vi "PM5000_VIF_demo_G2.vi"(2 "error in (no error)":errorcluster) -> (0 "error out":errorcluster, 1 "VIF_cluster":T1)   [LabVIEW 2018]
uses:
  Controls/VIF_cluster.ctl
panel:
  in  "Variacion Frecuencia":sgl=0.1
  in  "Variacion Voltaje":sgl=5.0
  in  "Frec_AVG":dbl=60.0
  in  "Frec.":dbl=60.0
  in  "I3":dbl=325.0
  in  "I2":dbl=320.0
  in  "I1":dbl=350.0
  in  "V3_V1":dbl=450.0
  in  "V2_V3":dbl=450.0
  in  "V1_V2":dbl=450.0
  # "VOLTAJES"
  # "CORRIENTE"
  # "FRECUENCIA"
  # "G02"
  # "G02"
  # "G02"
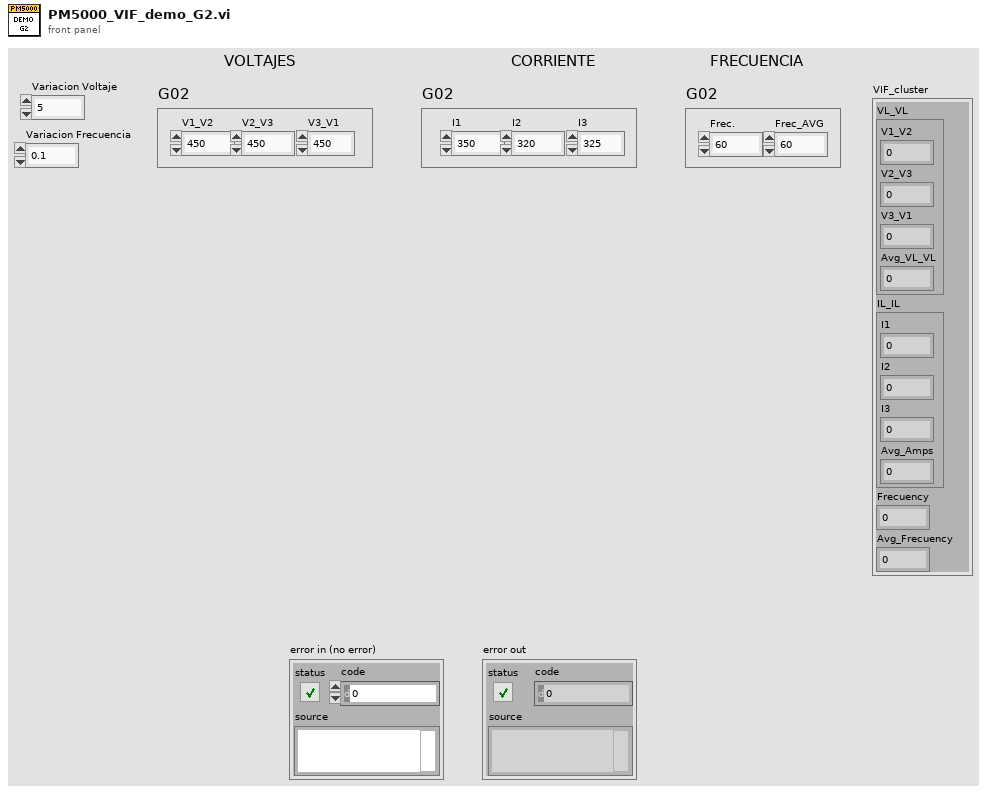
[diagram p1: front panel]
types:
  T1 = typedef "VIF_cluster.ctl" = cluster{"VL_VL":cluster{"V1_V2":sgl, "V2_V3":sgl, "V3_V1":sgl, "Avg_VL_VL":sgl}, "IL_IL":cluster{"I1":sgl, "I2":sgl, "I3":sgl, "Avg_Amps":sgl}, "Frecuency":sgl, "Avg_Frecuency":sgl}
  T2 = cluster{"I1 (A)":sgl, "I2 (A)":sgl, "I3 (A)":sgl, "Avg_Amps":sgl}
  T3 = cluster{"V1_V2 (V)":sgl, "V2_V3 (V)":sgl, "V3_V1 (V)":sgl, "Avg_VL_VL":sgl}
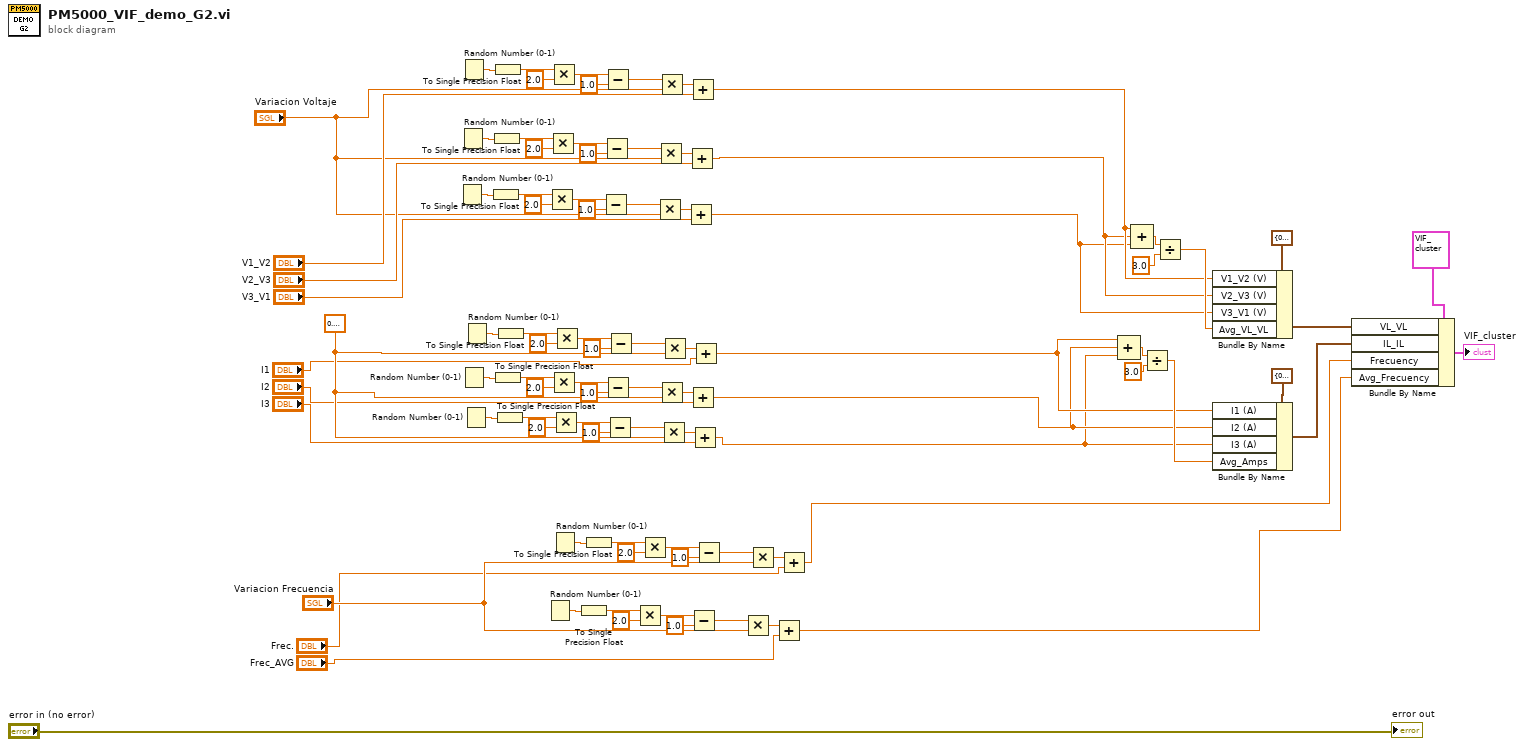
[diagram p0: block diagram]
diagram:
  w26 = sgl 0.1 ("y")
  n1 = Random Number (0-1)() -> (number: 0 to 1=w56:dbl)
  n2 = Random Number (0-1)() -> (number: 0 to 1=w64:dbl)
  n3 = Random Number (0-1)() -> (number: 0 to 1=w72:dbl)
  n4 = Random Number (0-1)() -> (number: 0 to 1=w37:dbl)
  n5 = Random Number (0-1)() -> (number: 0 to 1=w30:dbl)
  n6 = Random Number (0-1)() -> (number: 0 to 1=w44:dbl)
  n7 = To Single Precision Float(number=w56) -> (single precision float=w55:sgl)
  n8 = To Single Precision Float(number=w64) -> (single precision float=w65:sgl)
  n9 = To Single Precision Float(number=w72) -> (single precision float=w71:sgl)
  n10 = To Single Precision Float(number=w37) -> (single precision float=w36:sgl)
  n11 = To Single Precision Float(number=w30) -> (single precision float=w31:sgl)
  n12 = To Single Precision Float(number=w44) -> (single precision float=w45:sgl)
  n13 = Random Number (0-1)() -> (number: 0 to 1=w9:dbl)
  n14 = Multiply(x=w55, y=sgl 2.0) -> (x*y=w58:sgl)
  n15 = Multiply(x=w65, y=sgl 2.0) -> (x*y=w62:sgl)
  n16 = Multiply(x=w71, y=sgl 2.0) -> (x*y=w74:sgl)
  n17 = Multiply(x=w36, y=sgl 2.0) -> (x*y=w39:sgl)
  n18 = Random Number (0-1)() -> (number: 0 to 1=w16:dbl)
  n19 = Multiply(x=w31, y=sgl 2.0) -> (x*y=w28:sgl)
  n20 = Multiply(x=w45, y=sgl 2.0) -> (x*y=w42:sgl)
  n21 = To Single Precision Float(number=w9) -> (single precision float=w10:sgl)
  n22 = To Single Precision Float(number=w16) -> (single precision float=w15:sgl)
  n23 = Subtract(x=w58, y=sgl 1.0) -> (x-y=w54:sgl)
  n24 = Subtract(x=w62, y=sgl 1.0) -> (x-y=w66:sgl)
  n25 = Subtract(x=w74, y=sgl 1.0) -> (x-y=w70:sgl)
  n26 = Subtract(x=w39, y=sgl 1.0) -> (x-y=w35:sgl)
  n27 = Subtract(x=w28, y=sgl 1.0) -> (x-y=w32:sgl)
  n28 = Subtract(x=w42, y=sgl 1.0) -> (x-y=w46:sgl)
  n29 = Multiply(x=w10, y=sgl 2.0) -> (x*y=w7:sgl)
  n30 = Multiply(x=w15, y=sgl 2.0) -> (x*y=w18:sgl)
  n31 = Multiply(x=w54, y="Variacion Voltaje") -> (x*y=w53:sgl)
  n32 = Multiply(x=w66, y="Variacion Voltaje") -> (x*y=w67:sgl)
  n33 = Multiply(x=w70, y="Variacion Voltaje") -> (x*y=w69:sgl)
  n34 = Multiply(x=w35, y=w26) -> (x*y=w34:sgl)
  n35 = Multiply(x=w32, y=w26) -> (x*y=w33:sgl)
  n36 = Multiply(x=w46, y=w26) -> (x*y=w47:sgl)
  n37 = Add(x=w53, y="V3_V1") -> (x+y=w48:dbl)
  n38 = Add(x=w67, y="V2_V3") -> (x+y=w49:dbl)
  n39 = Add(x=w69, y="V1_V2") -> (x+y=w50:dbl)
  n40 = Add(x=w34, y="I2") -> (x+y=w21:dbl)
  n41 = Subtract(x=w7, y=sgl 1.0) -> (x-y=w11:sgl)
  n42 = Add(x=w33, y="I3") -> (x+y=w20:dbl)
  n43 = Add(x=w47, y="I1") -> (x+y=w22:dbl)
  n44 = Subtract(x=w18, y=sgl 1.0) -> (x-y=w14:sgl)
  n45 = Multiply(x=w11, y="Variacion Frecuencia") -> (x*y=w12:sgl)
  n46 = Multiply(x=w14, y="Variacion Frecuencia") -> (x*y=w13:sgl)
  n47 = Add(x=w12, y="Frec_AVG") -> (x+y=w3:dbl)
  n48 = Add(x=w13, y="Frec.") -> (x+y=w4:dbl)
  n49 = Compound Arithmetic op=ADD(w22, w21, w20) -> (w77:dbl)
  n50 = Compound Arithmetic op=ADD(w50, w49, w48) -> (w81:dbl)
  n51 = Divide(x=w77, y=sgl 3.0) -> (x/y=w76:dbl)
  n52 = Divide(x=w81, y=sgl 3.0) -> (x/y=w79:dbl)
  n53 = Bundle By Name(cluster=T3 {"V1_V2 (V)"=0.0, "V2_V3 (V)"=0.0, "V3_V1 (V)"=0.0, "Avg_VL_VL"=0.0} ("VL_VL"), "V1_V2 (V)"=w50, "V2_V3 (V)"=w49, "V3_V1 (V)"=w48, "Avg_VL_VL"=w79) -> (w84:T3)
  n54 = Bundle By Name(cluster=T2 {"I1 (A)"=0.0, "I2 (A)"=0.0, "I3 (A)"=0.0, "Avg_Amps"=0.0} ("IL_IL"), "I1 (A)"=w22, "I2 (A)"=w21, "I3 (A)"=w20, "Avg_Amps"=w76) -> (w83:T2)
  n55 = Bundle By Name(cluster=T1 {"VL_VL"={"V1_V2"=0.0, "V2_V3"=0.0, "V3_V1"=0.0, "Avg_VL_VL"=0.0}, "IL_IL"={"I1"=0.0, "I2"=0.0, "I3"=0.0, "Avg_Amps"=0.0}, "Frecuency"=0.0, "Avg_Frecuency"=0.0} ("VIF_cluster"), "VL_VL"=w84, "IL_IL"=w83, "Frecuency"=w4, "Avg_Frecuency"=w3) -> (→"VIF_cluster":T1)
  "error out" <- "error in (no error)"
